vi "Stop Trial.vi"(8 "error in (no error)":errorcluster, 9 "DAQ Task":bool, 10 "Stop Acquiring":bool, 11 "NI Force Task in":refnum<class "NI Force Task.lvclass">) -> (0 "error out":errorcluster, 3 "NI Force Task out":refnum<class "NI Force Task.lvclass">)   [LabVIEW 2020, in "NI Force Task.lvlib" / "NI Force Task.lvclass"]
uses:
  NI Force Task.lvclass
  NI Force Task.lvclass/NI Force Task.ctl
  Lissajous Viewer Messages/Start Stop Trial Msg/Start Stop Trial Msg.lvclass
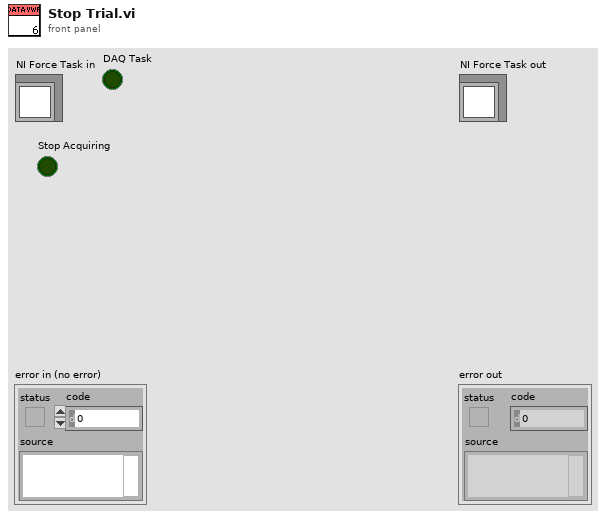
[diagram p1: front panel]
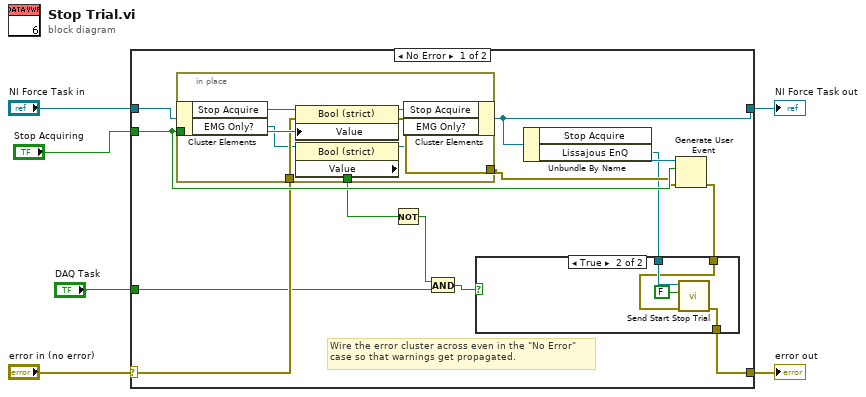
[diagram p0: block diagram]
diagram:
  n1 = case shown="No Error" "error in (no error)" {
    selector: "error in (no error)" -> [w14 w34]
    tunnel: [w11 w34] -> w5
    tunnel: [w18 w33] -> w3
    tunnel: "NI Force Task in" -> [w19 w33]
    tunnel: "Stop Acquiring" -> [w16 _]
    tunnel: "DAQ Task" -> [w10 _]
    frame No Error {
      # "Wire the error cluster across even in the \"No Error\"\ncase so that warnings get propagated."
      n2 = in-place {
        in-place-border: w16 -> [w30]
        in-place-border: w14 -> [w29]
        in-place-border: [w28] -> w15
        in-place-border: [w25] -> w8
        n3 = in-place-cluster #1(w19) -> ("Stop Acquire"=w32:refnum<vi>, "EMG Only?"=w27:refnum<vi>)
        n4 = property class="Bool (strict)"(reference=w32, error in=w29, "Value"=w30) -> (reference out=w31:refnum<vi>, error out=w28:errorcluster)
        n5 = property class="Bool (strict)"(reference=w27) -> (reference out=w26:refnum<vi>, "Value"=w25:bool)  [unwired: 1 in, 1 out]
        n6 = in-place-cluster #1("Stop Acquire"=w31, "EMG Only?"=w26) -> (w18:refnum<class "NI Force Task.lvclass">)
      }
      n7 = Not(x=w8) -> (.not. x?=w7:bool)
      n8 = And(x=w7, y=w10) -> (x .and. y?=w9:bool)
      n9 = Unbundle By Name(w18) -> ("Stop Acquire"=w17:refnum<user-event>, "Lissajous EnQ"=w13:refnum<class "Message Enqueuer.lvclass">)
      n10 = Generate User Event(user event=w17, event data cluster=w16, error in=w15) -> (error out=w12:errorcluster)  [unwired: 1 in, 1 out]
      n11 = case shown="True" w9 {
        tunnel: w13 -> [_ w24]
        tunnel: w12 -> [w20 w23]
        tunnel: [w20 w22] -> w11
        frame False {
        }
        frame True {
          n12 = call "Send Start Stop Trial.vi"("error in (no error)"=w23, "Acquiring true?"=FALSE, "Message Enqueuer in"=w24) -> ("error out"=w22:errorcluster)  [unwired: 7 in, 1 out]
        }
      }
    }
    frame Error {
    }
  }
  "error out" <- w5
  "NI Force Task out" <- w3
